vi "Get n Days before Time string.vi"(8 "error in (no error)":errorcluster, 11 "Days":u32) -> (0 "error out":errorcluster, 1 "23:59:59":string, 2 "00:00:00":string, 3 "n days before Current time string":string, 5 "n days before Current time stamp":timestamp)   [LabVIEW 2021]
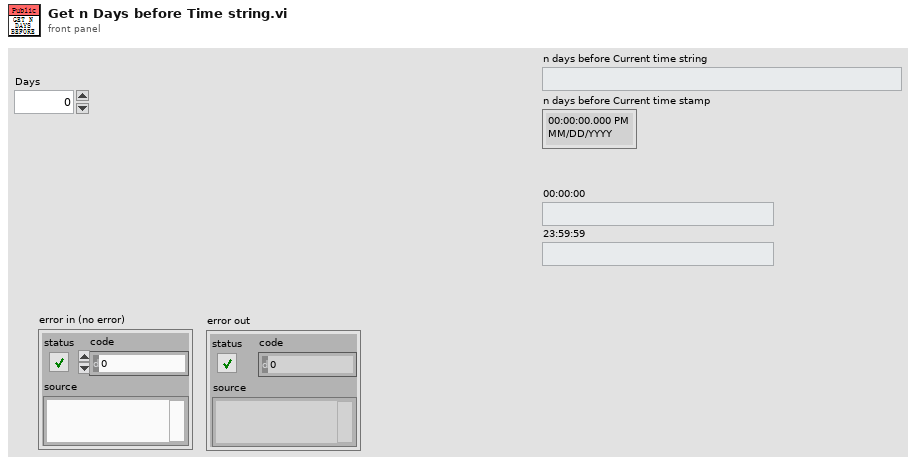
[diagram p1: front panel]
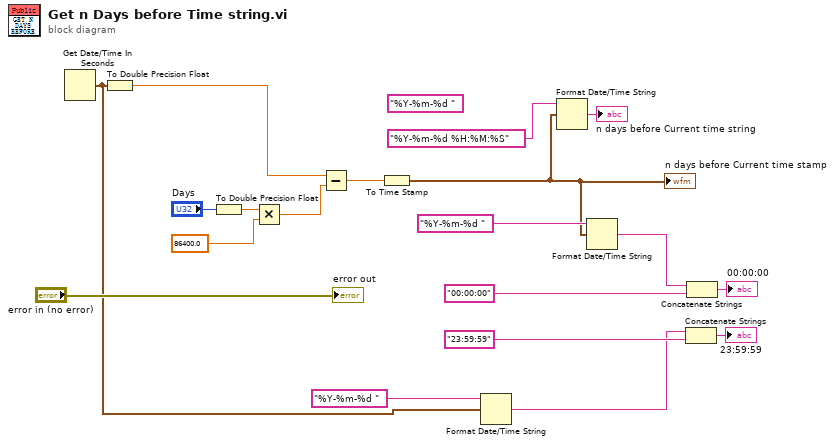
[diagram p0: block diagram]
diagram:
  (unwired) "%Y-%m-%d " ("time format string (%c)")
  n1 = Get Date/Time In Seconds() -> (seconds since 1Jan1904=w4:timestamp)
  n2 = To Double Precision Float(number=w4) -> (double precision float=w16:dbl)
  n3 = To Double Precision Float(number="Days") -> (double precision float=w17:dbl)
  n4 = Multiply(x=w17, y=86400.0) -> (x*y=w15:dbl)
  n5 = Subtract(x=w16, y=w15) -> (x-y=w14:dbl)
  n6 = To Time Stamp(1:w14) -> (0:w9:timestamp)
  "n days before Current time stamp" <- w9
  n7 = Format Date/Time String(time format string (%c)="%Y-%m-%d ", seconds (now)=w4) -> (date/time string=w3:string)  [unwired: 1 in]
  n8 = Format Date/Time String(time format string (%c)="%Y-%m-%d %H:%M:%S", seconds (now)=w9) -> (date/time string=→"n days before Current time string":string)  [unwired: 1 in]
  n9 = Format Date/Time String(time format string (%c)="%Y-%m-%d ", seconds (now)=w9) -> (date/time string=w2:string)  [unwired: 1 in]
  n10 = Concatenate Strings(w3, "23:59:59" ("Numeric Text.Text 2")) -> (→"23:59:59":string)
  n11 = Concatenate Strings(w2, "00:00:00" ("Numeric Text.Text 2")) -> (→"00:00:00":string)
  "error out" <- "error in (no error)"
